vi "Admittance_control_27_07_2017.vi"() -> ()   [LabVIEW 2016]
uses:
  <vilib>/Platform/TimedLoop/XDataNode/timing_clust.ctl
  <vilib>/Platform/TimedLoop/XDataNode/nitl_modes.ctl
  <vilib>/Platform/TimedLoop/XDataNode/wakeup.ctl
  <vilib>/Platform/TimedLoop/XDataNode/loadnilvce.vi
  <vilib>/Motion/Express/_s/nimc.ax.power.power.axis.vi
  <vilib>/Motion/Express/_s/nimc.fb.read.readExecutionData.axis.vi
  <vilib>/Motion/Express/_s/nimc.fb.stopMove.stop.axis.modeDecelerate.vi
  <vilib>/Motion/Express/_s/nimc.fb.straightLineMove.startStraightLineMove.axis.modeVelocity.0.vi
  <vilib>/Motion/Express/_s/nimc.fb.resetPosition.resetPosition.axis.vi
  <vilib>/Motion/Express/_s/nimc.ex.power.power.axis.vi
  <vilib>/platform/TimedLoop/XDataNode/XDataNode.xnode
  <vilib>/Motion/BlockNode/FB.NIMotion.xnode
  <vilib>/Platform/TimedLoop/XDataNode/XDNodeRunTimeDep.lvlib
panel:
  in  "Speed gain":dbl=0.25 format="%#_12g"
  in  "Torque limit  2":dbl=0.25 format="%#_12g"
  out "Boolean 7":bool
  out "Boolean 6":bool
  in  "Torque limit":dbl=0.25 format="%#_12g"
  out "Boolean 5":bool
  out "Boolean 4":bool
  out "Boolean 3":bool
  out "post sin 2":dbl format="%#_13g"
  out "motor torque, Nm 2":dbl format="%.3f"
  out "Torque 2":dbl(knob) scale=-1.0..2.0
  out "post sin":dbl format="%#_13g"
  out "pre sin":dbl format="%#_13g"
  out "Adjusted Motor Velocity":dbl format="%.3f"
  out "Adjusted Velocity":dbl(knob) scale=-1.0..2.0
  in  "Reset Position":bool
  in  "Speed":dbl=0.25 format="%#_12g"
  out "Torque":dbl(knob) scale=-3.0..3.0
  out "Position":dbl(knob) scale=-1.0..1.0
  out "Velocity":dbl(knob) scale=-1.0..5.0
  out "Load Cell":dbl(knob) scale=0.0..10.0
  in  "Move to Position?":bool
  out "Load cell, V":dbl format="%.3f"
  out "motor torque, Nm":dbl format="%.3f"
  out "motor velocity, rev/s":dbl format="%.3f"
  out "motor position, rev":dbl format="%.3f"
  in  "STOP VI":bool
  in  "Enable Axis \nControl":bool
  in  "Enable Motor \nDrive":bool
  in  "EMERGENCY MOTOR STOP":bool
  # "Raw Data from System"
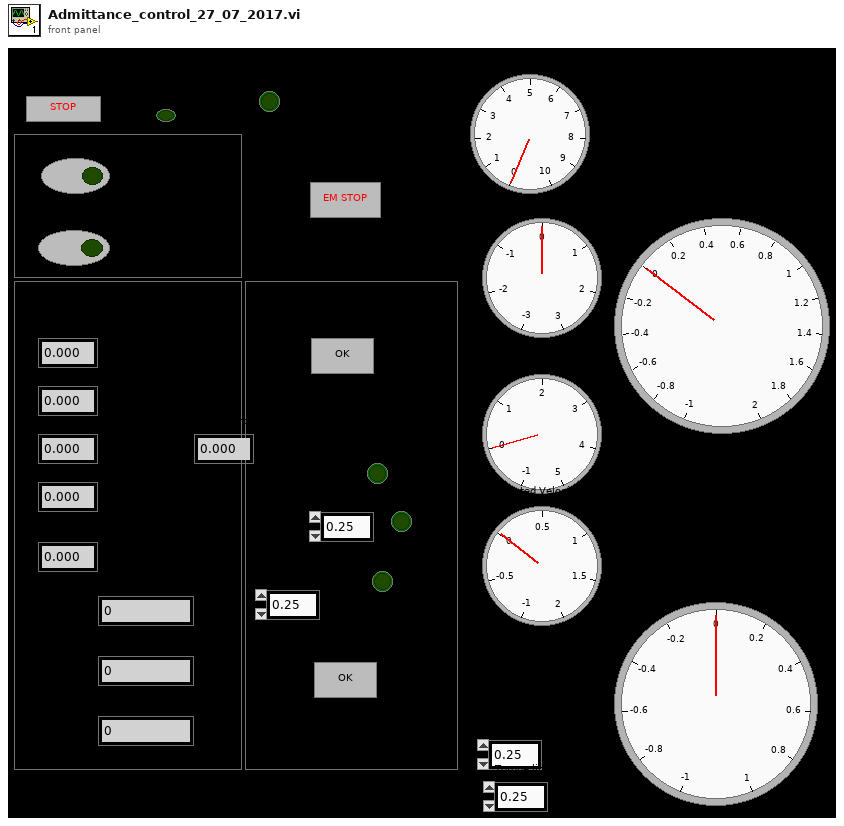
[diagram p1: front panel]
types:
  T1 = typedef "XDNodeRunTimeDep.lvlib/timing_clust.ctl" = cluster{"Expected End [f-1]":u64, "Actual End [f-1]":u64, "Finished Late? [f-1]":bool, "Expected End [i-1]":u64, "Actual End [i-1]":u64, "Finished Late? [i-1]":bool, "Expected Start [i]":u64, "Actual Start [i]":u64, "Expected Start [f]":u64, "Actual Start [f]":u64, "Source Name":string, "Structure Name":string, "Period":i64, "Deadline":i64, "Offset":i64, "Start":i64, "Priority":i32, "Timeout":i32, "Mode":T2, "Wakeup Reason":T3, "Error":errorcluster, "Source Type":string, "Secondary Source Type":string, "Global End Time":u64, "Global Start Time":u64, "Frame Duration":u64, "Iteration Duration":u64, "Assigned CPU":i32, "I/O Scan Engine Mode":u32}
  T2 = typedef "XDNodeRunTimeDep.lvlib/nitl_modes.ctl" = enum32{"No Change", "Process missed periods, maintain original phase", "Discard missed periods, maintain original phase", "Process missed periods, ignore original phase", "Discard missed periods, ignore original phase"}
  T3 = typedef "XDNodeRunTimeDep.lvlib/wakeup.ctl" = enum32{"Normal", "Aborted", "Asynchronous wakeup", "Timing source error", "Timed loop error", "Timeout"}
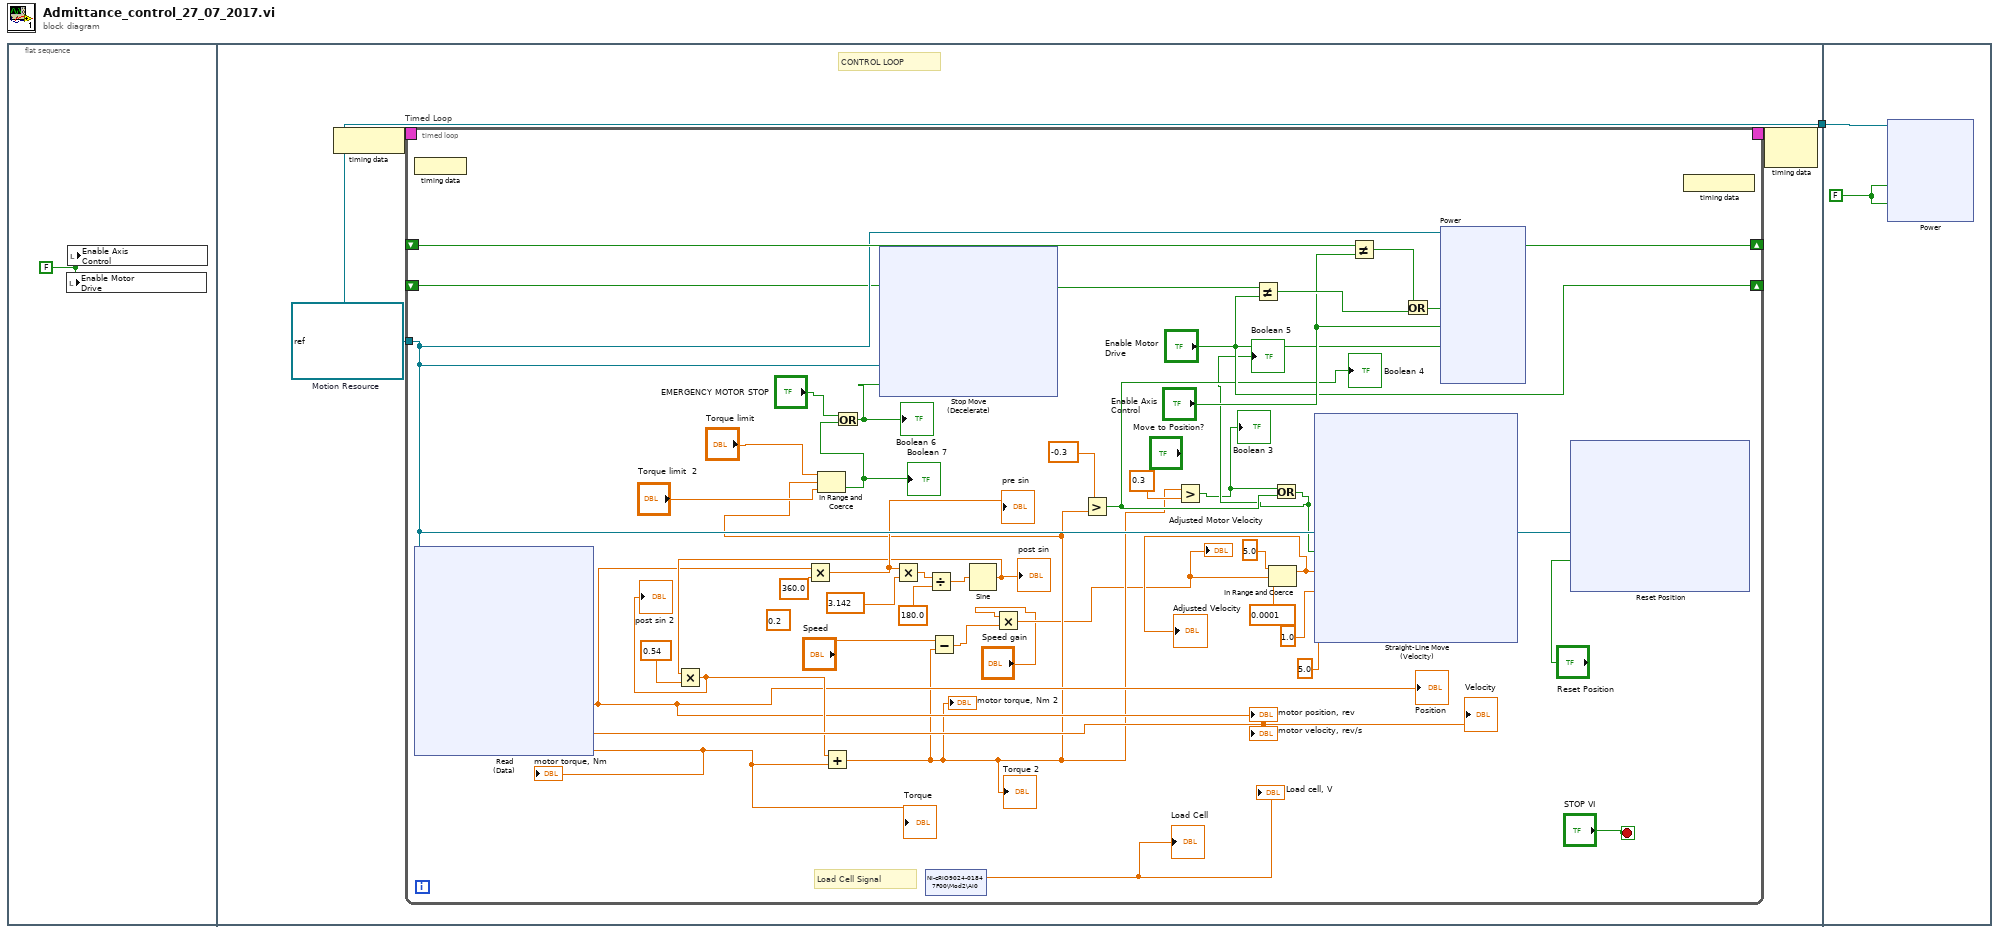
[diagram p0: block diagram]
diagram:
  n1 = flat-sequence {
    tunnel: [w5] -> w1
    tunnel: w1 -> [w127]
    frame #0 {
      w2 = FALSE
      n2 = local write "Enable Motor \nDrive"(w2) -> ()
      n3 = local write "Enable Axis \nControl"(w2) -> ()
    }
    frame #1 {
      w5 = refnum<k21> "nism://NI-cRIO9024-01847F00/Axis 1"  # Motion Resource
      # "CONTROL LOOP"
      n4 = node-c288() -> (w4:T1)
      n5 = timed-loop "Timed Loop" {
        tunnel: w5 -> [w41]
        timing: w4 -> [_]
        timing-out: [_] -> w3
        shift-right: ["Enable Axis \nControl"] -> _
        shift-left: _ -> [w48]
        shift-right: ["Enable Motor \nDrive"] -> _
        shift-left: _ -> [w35]
        stop <- "STOP VI" stop-if-true
        (unwired) 0.2
        # "Load Cell Signal"
        n6 = node-c288() -> ()  [unwired: 1 in]
        n7 = xnode "Read\n(Data)"("resource"=w41) -> ("position"=w19:dbl, "torque"=w22:dbl, "velocity"=→"motor velocity, rev/s" →"Velocity":dbl)  [unwired: 1 in, 3 out]
        "motor position, rev" <- w19
        "motor torque, Nm" <- w22
        "Position" <- w19
        "Torque" <- w22
        n8 = Multiply(x=w19, y=360.0) -> (x*y=w33:dbl)
        "pre sin" <- w33
        n9 = Multiply(x=w33, y=3.142) -> (x*y=w31:dbl)
        n10 = shared-variable "NI-cRIO9024-01847F00\\Mod2\\AI0"() -> (→"Load cell, V" →"Load Cell":dbl)  [unwired: 1 in, 1 out]
        n11 = Divide(x=w31, y=180.0) -> (x/y=w30:dbl)
        n12 = Sine(x=w30) -> (sin(x)=w23:dbl)
        "post sin" <- w23
        n13 = Multiply(x=w23, y=0.54) -> (x*y=w21:dbl)
        "post sin 2" <- w21
        n14 = Add(x=w21, y=w22) -> (x+y=w9:dbl)
        "Torque 2" <- w9
        "motor torque, Nm 2" <- w9
        n15 = In Range and Coerce(upper limit="Torque limit", x=w9, lower limit="Torque limit  2") -> (In Range?=w11:bool)  [unwired: 1 out]
        "Boolean 7" <- w11
        n16 = Or(x="EMERGENCY MOTOR STOP", y=w11) -> (x .or. y?=w13:bool)
        "Boolean 6" <- w13
        n17 = xnode "Stop Move\n(Decelerate)"("resource"=w41, "execute"=w13) -> ()  [unwired: 1 in, 3 out]
        n18 = Subtract(x="Speed", y=w9) -> (x-y=w7:dbl)
        n19 = Multiply(x="Speed gain", y=w7) -> (x*y=w8:dbl)
        "Adjusted Motor Velocity" <- w8
        n20 = Greater?(x=-0.3, y=w9) -> (0:w17:bool)
        "Boolean 4" <- w17
        n21 = Greater?(x=w9, y=0.3) -> (0:w15:bool)
        "Boolean 3" <- w15
        n22 = Not Equal?(x=w35, y="Enable Motor \nDrive") -> (x != y?=w46:bool)
        n23 = In Range and Coerce(upper limit=5.0, x=w8, lower limit=0.0001) -> (coerced(x)=w26:dbl)  [unwired: 1 out]
        "Adjusted Velocity" <- w26
        n24 = Or(x=w15, y=w17) -> (x .or. y?=w16:bool)
        "Boolean 5" <- w16
        n25 = xnode "Straight-Line Move\n(Velocity)"("resource"=w41, "execute"=w16, "velocity"=w26, "acceleration"=1.0, "deceleration"=5.0) -> ("resource out"=w38:refnum<k21>)  [unwired: 1 in, 2 out]
        n26 = Not Equal?(x=w48, y="Enable Axis \nControl") -> (x != y?=w47:bool)
        n27 = Or(x=w47, y=w46) -> (x .or. y?=w45:bool)
        n28 = xnode ("Power")("execute"=w45, "enable axis"="Enable Axis \nControl", "enable drive"="Enable Motor \nDrive", "resource"=w41) -> ()  [unwired: 1 in, 6 out]
        n29 = xnode "Reset Position"("resource"=w38, "execute"="Reset Position") -> ()  [unwired: 2 in, 3 out]
        n30 = node-c288() -> ()  [unwired: 1 out]
      }
      n31 = node-c288(w3) -> ()  [unwired: 1 out]
    }
    frame #2 {
      w128 = FALSE
      n32 = xnode ("Power")("enable axis"=w128, "enable drive"=w128, "resource"=w127) -> ()  [unwired: 1 in, 2 out]
    }
  }
